vi "GetAllMethodsTypesForClass.vi"(0 "ClassWriterNative":refnum<class "ClassWriterNative.lvclass">, 5 "ClassItemRefIn":refnum<vi>, 11 "error in":errorcluster) -> (2 "MethodTemplatePathOut":path, 3 "DesignPattern":T4[](array[typedef]), 4 "NormalMethods":T2[](array[typedef]), 6 "OverrideMethods":T2[](array[typedef]), 8 "PropertyMethods":T2[](array[typedef]), 10 "ConnectorPaneHeight":i32[](array[numeric]), 13 "TemplateSettings":T1, 14 "PropertyNodeMethods":T2[](array[typedef]), 15 "error out":errorcluster)   [LabVIEW 2012, in "ClassWriterNative.lvclass"]
uses:
  <resource>/Framework/Providers/Open_GDS/ClassProviders/Provider_LvNativeClass/ClassWriterNative_class/ClassWriterNative.lvclass
  <resource>/Framework/Providers/Open_GDS/ClassProviders/Provider_LvNativeClass/ClassWriterNative_class/MethodInfo.ctl
  <resource>/Framework/Providers/Open_GDS/ClassProviders/Provider_LvNativeClass/ClassWriterNative_class/MethodType.ctl
  <resource>/Framework/Providers/Open_GDS/ClassProviders/Common/LvClass_class/GDSLvClass_PlugIn.ctl
  <resource>/Framework/Providers/Open_GDS/ClassProviders/Common/LvClass_class/GDSLvClass_PlugInTypes.ctl
  <resource>/Framework/Providers/Open_GDS/ClassProviders/Provider_BaseClassInterface/ClassWriter_class/TemplateSettings.ctl
  <resource>/Framework/Providers/Open_GDS/ClassProviders/Provider_BaseClassInterface/BaseProvider_SubVIs/BaseProvider_PlugInManagerActions.ctl
  <resource>/Framework/Providers/Open_GDS/ClassProviders/Provider_BaseClassInterface/ClassWriter_class/ClassWriter.lvclass
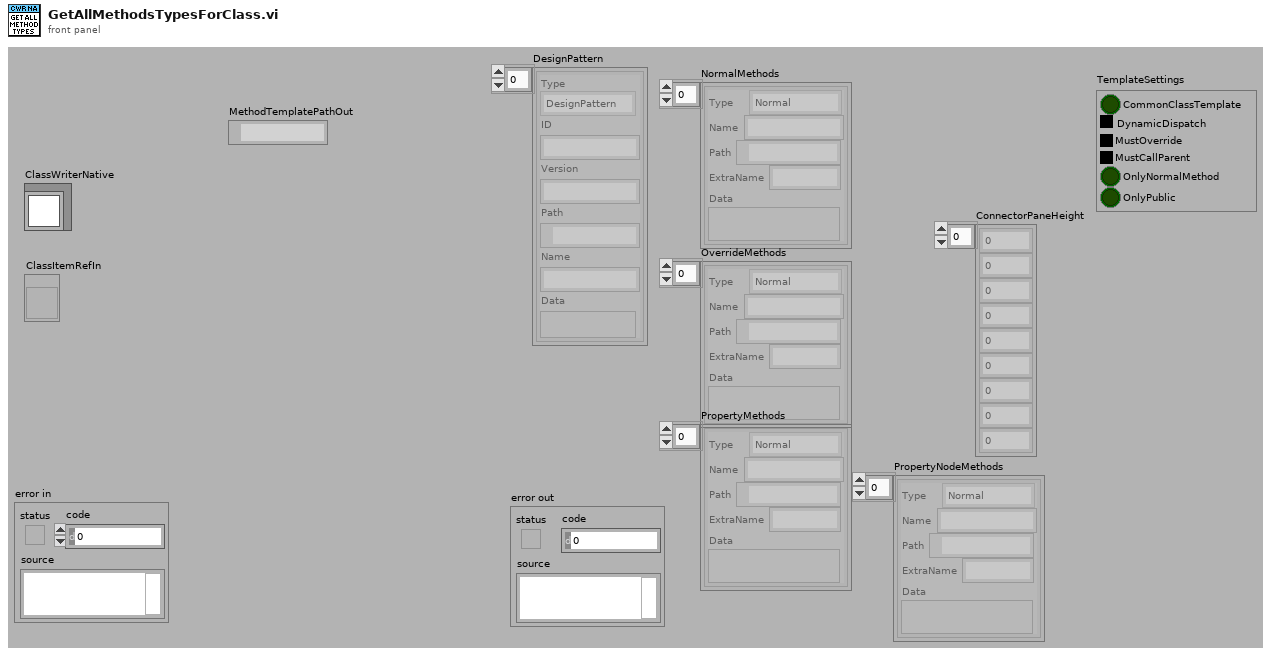
[diagram p1: front panel]
types:
  T1 = typedef "ClassWriter.lvclass/TemplateSettings.ctl" = cluster{"CommonClassTemplate":bool, "DynamicDispatch":enum8{"False", "True", "Mixed"}, "MustOverride":enum8{"False", "True", "Mixed"}, "MustCallParent":enum8{"False", "True", "Mixed"}, "OnlyNormalMethod":bool, "OnlyPublic":bool}
  T2 = typedef "ClassWriterNative.lvclass/MethodInfo.ctl" = cluster{"Type":T3, "Name":string, "Path":path, "ExtraName":string, "Data":variant}
  T3 = typedef "ClassWriterNative.lvclass/MethodType.ctl" = enum16{"Normal", "MethodPlugIn", "DesignPattern", "AF-Method"}
  T4 = typedef "GDSLvClass_PlugIn.ctl" = cluster{"Type":T5, "ID":string, "Version":string, "Path":path, "Name":string, "Data":variant}
  T5 = typedef "GDSLvClass_PlugInTypes.ctl" = enum16{"DesignPattern", "MethodTypes"}
  T6 = typedef "GDSLvCLass_ClassSettingsType.ctl" = cluster{"ClassProviderName":string, "ClassTemplateUsed":string, "ClassTemplateVersion":string, "ClassDescription":string, "PlugIns":T4[], "ConnectorPanePattern":string}
  T7 = typedef "BaseProvider_PlugInManagerActions.ctl" = enum16{"GetPluginsMethods", "ExecutePlugIn"}
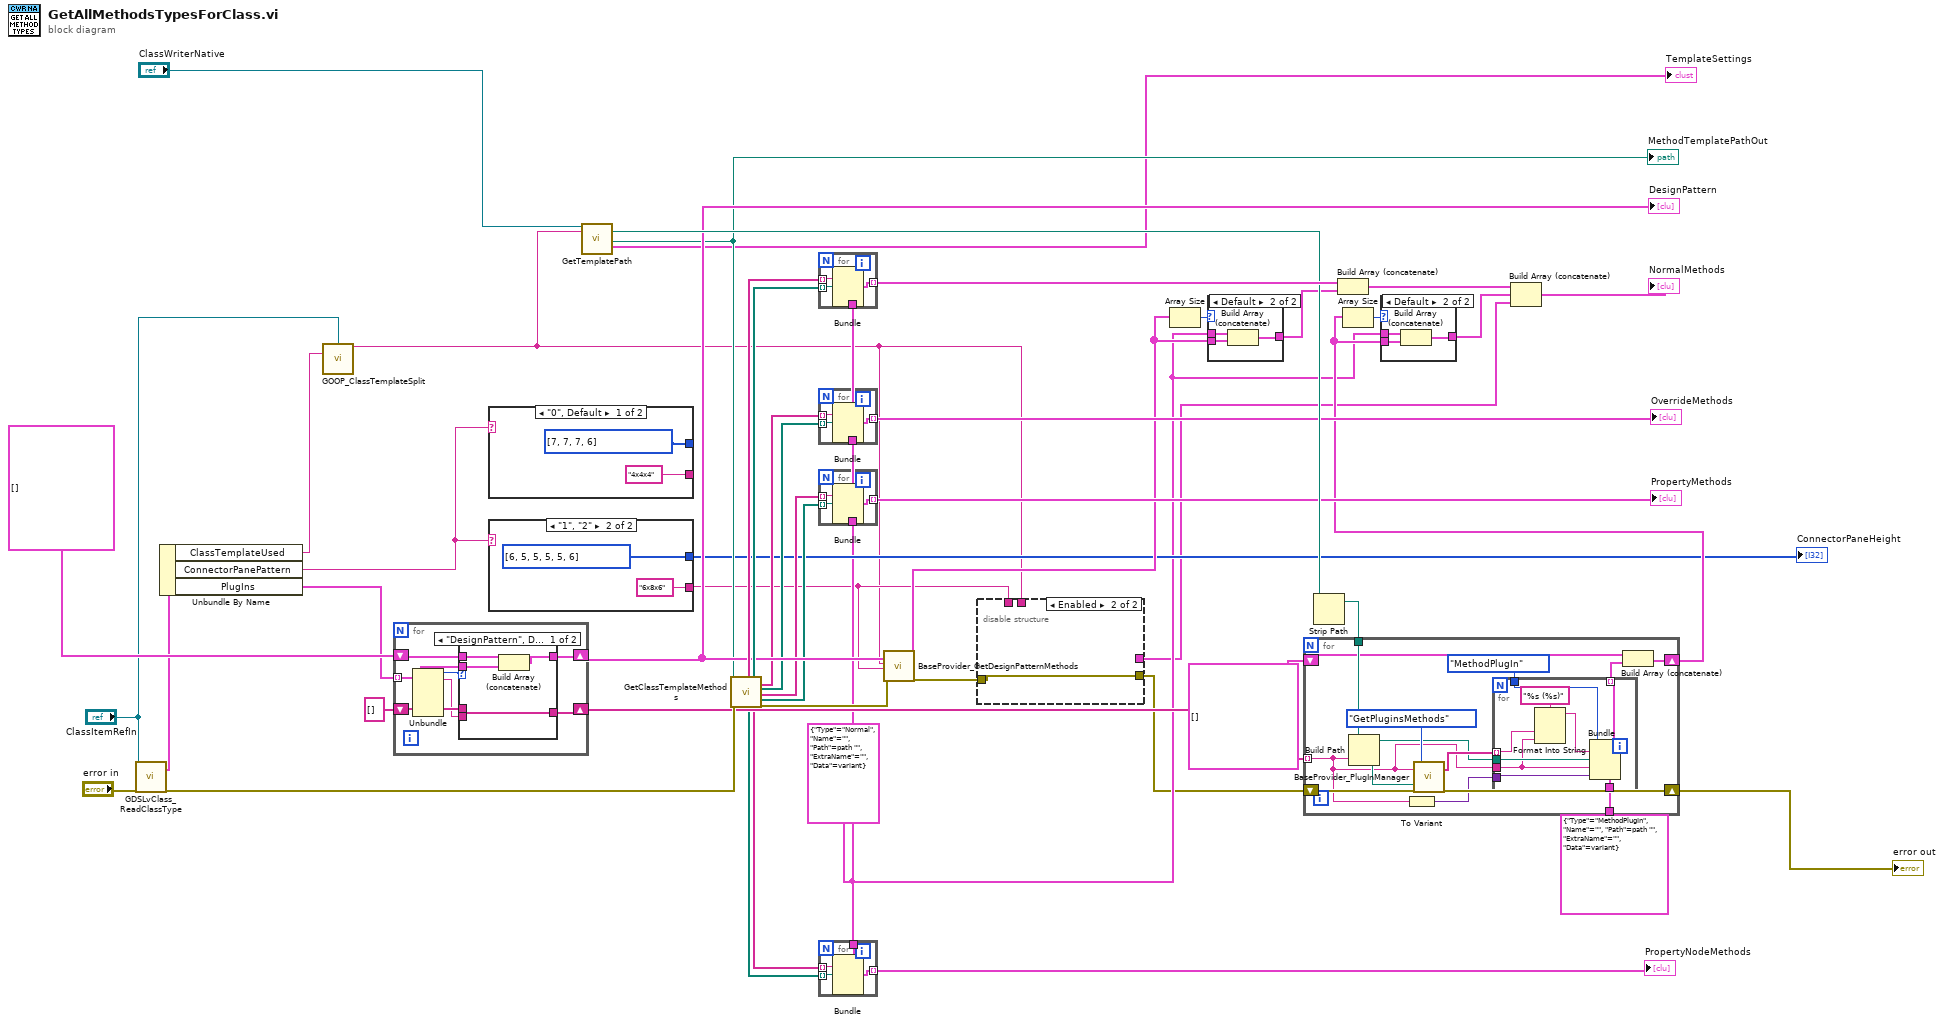
[diagram p0: block diagram]
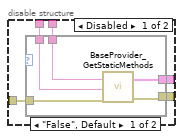
[diagram p2: hidden frame]
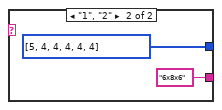
[diagram p4: hidden frame]
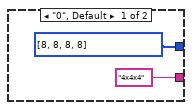
[diagram p5: hidden frame]
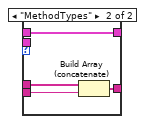
[diagram p8: hidden frame]
diagram:
  w10 = T2 {"Type"=enum."Normal", "Name"="", "Path"=path "", "ExtraName"="", "Data"=variant} ("Cluster")
  n1 = call <resource>:"GDSLvClass_ReadClassType.vi"("Class Refnum In"="ClassItemRefIn", "error in (no error)"="error in") -> ("ClassSettings"=w33:T6, "error out"=w46:errorcluster)  [unwired: 15 in, 1 out]
  n2 = Unbundle By Name(w33) -> ("ClassTemplateUsed"=w13:string, "ConnectorPanePattern"=w12:string, "PlugIns"=w35:T4[])
  n3 = call <resource>:"GOOP_ClassTemplateSplit.vi"("ClassItemRefIn"="ClassItemRefIn", "FullClassTemplate"=w13) -> ("StandardTemplate"=w2:string)  [unwired: 12 in, 1 out]
  n4 = for {
    tunnel: w35 -> [w48] mode=indexing
    shift-right: [w52] -> w41
    shift-left: string[] [] -> [w53]
    shift-right: [w49] -> w37
    shift-left: T4[] [] -> [w50]
    n5 = Unbundle(w48) -> ("Type"=w54:T5, "ID"=w51:string)  [unwired: 4 out]
    n6 = case shown="\"DesignPattern\", Default" w54 {
      tunnel: w53 -> [w58 w62]
      tunnel: [w58 w61] -> w52
      tunnel: w51 -> [_ w60]
      tunnel: w50 -> [w57 w59]
      tunnel: [w56 w59] -> w49
      tunnel: w48 -> [w55 _]
      frame "DesignPattern", Default {
        n7 = Build Array (concatenate)(w57, w55) -> (w56:T4[])
      }
      frame "MethodTypes" {
        n8 = Build Array (concatenate)(w62, w60) -> (w61:string[])
      }
    }
  }
  "DesignPattern" <- w37
  n9 = case shown="\"0\", Default" w12 {
    tunnel: ["4x4x4" "6x8x6"] -> _
    tunnel: [i32[] [7, 7, 7, 6] ("ConnectorPaneHeight") i32[] [5, 4, 4, 4, 4, 4] ("ConnectorPaneHeight")] -> _
    frame "0", Default {
    }
    frame "1", "2" {
    }
  }
  n10 = case shown="\"1\", \"2\"" w12 {
    tunnel: ["4x4x4" "6x8x6"] -> w3
    tunnel: [i32[] [8, 8, 8, 8] ("ConnectorPaneHeight") i32[] [6, 5, 5, 5, 5, 6] ("ConnectorPaneHeight")] -> w14
    frame "0", Default {
    }
    frame "1", "2" {
    }
  }
  "ConnectorPaneHeight" <- w14
  n11 = call-dynamic "GetTemplatePath.vi"("reference in"="ClassWriterNative", "ClassTemplateSubDirectory"=w2) -> ("FolderPathOut"=w39:path, "MethodTemplatePathOut"=w24:path, "TemplateSettings"=→"TemplateSettings":T1)  [unwired: 13 in, 2 out]
  "MethodTemplatePathOut" <- w24
  n12 = call <resource>:"GetClassTemplateMethods.vi"("MethodTemplatePath"=w24, "error in"=w46) -> ("NormalMethodNames"=w42:string[], "PropertyNodeMethodPaths"=w8:path[], "NormalMethodPaths"=w43:path[], "PropertyNodeMethodNames"=w9:string[], "OverrideMethodNames"=w32:string[], "OverrideMethodPaths"=w31:path[], "PropertyMethodNames"=w29:string[], "PropertyMethodPaths"=w28:path[], "error out"=w47:errorcluster)  [unwired: 9 in]
  n13 = for {
    tunnel: w42 -> [w73] mode=indexing
    tunnel: w43 -> [w72] mode=indexing
    tunnel: w10 -> [w74]
    tunnel: [w71] -> w44 mode=indexing
    n14 = Bundle(cluster=w74, "Name"=w73, "Path"=w72) -> (w71:T2)  [unwired: 3 in]
  }
  n15 = for {
    tunnel: w32 -> [w77] mode=indexing
    tunnel: w31 -> [w76] mode=indexing
    tunnel: w10 -> [w78]
    tunnel: [w75] -> w30 mode=indexing
    n16 = Bundle(cluster=w78, "Name"=w77, "Path"=w76) -> (w75:T2)  [unwired: 3 in]
  }
  "OverrideMethods" <- w30
  n17 = for {
    tunnel: w29 -> [w81] mode=indexing
    tunnel: w28 -> [w80] mode=indexing
    tunnel: w10 -> [w82]
    tunnel: [w79] -> w27 mode=indexing
    n18 = Bundle(cluster=w82, "Name"=w81, "Path"=w80) -> (w79:T2)  [unwired: 3 in]
  }
  "PropertyMethods" <- w27
  n19 = for {
    tunnel: w9 -> [w85] mode=indexing
    tunnel: w8 -> [w84] mode=indexing
    tunnel: w10 -> [w86]
    tunnel: [w83] -> w7 mode=indexing
    n20 = Bundle(cluster=w86, "Name"=w85, "Path"=w84) -> (w83:T2)  [unwired: 3 in]
  }
  "PropertyNodeMethods" <- w7
  n21 = call <resource>:"BaseProvider_GetDesignPatternMethods.vi"("DesignPattern"=w37, "ClassTemplateName"=w2, "ConnectorPaneSettings"=w3, "error in"=w47) -> ("NormalMethods"=w16:T2[], "error out"=w6:errorcluster)  [unwired: 14 in]
  n22 = disable-structure shown="Enabled" {
    disable-tunnel: w6 -> [w91 w98]
    disable-tunnel: [w90 w98] -> w5
    disable-tunnel: [w89 _] -> w4
    disable-tunnel: w3 -> [w88 _]
    disable-tunnel: w2 -> [w87 _]
    frame Disabled {
      n23 = case shown="\"False\", Default" {
        selector: _ -> [_ _]
        tunnel: w91 -> [w96 w97]
        tunnel: [w95 w97] -> w90
        tunnel: [w94 _] -> w89
        tunnel: w88 -> [w93 _]
        tunnel: w87 -> [w92 _]
        frame "False", Default {
          n24 = call <resource>:"BaseProvider_GetStaticMethods.vi"("ClassTemplateName"=w92, "ConnectorPaneSettings"=w93, "error in"=w96) -> ("NormalMethods"=w94:T2[], "error out"=w95:errorcluster)  [unwired: 15 in]
        }
        frame "True" {
        }
      }
    }
    frame Enabled {
    }
  }
  n25 = Array Size(array=w16) -> (size(s)=w26:i32)
  n26 = case shown="Default" w26 {
    tunnel: w16 -> [w99 w102]
    tunnel: [w99 w101] -> w25
    tunnel: w10 -> [_ w100]
    frame 0 {
    }
    frame Default {
      n27 = Build Array (concatenate)(w100, w102) -> (w101:T2[])
    }
  }
  n28 = Strip Path(path=w39) -> (stripped path=w40:path)  [unwired: 1 out]
  n29 = for {
    shift-right: [w114] -> w45
    shift-left: w5 -> [w113]
    tunnel: w41 -> [w103] mode=indexing
    tunnel: w40 -> [w112]
    shift-right: [w110] -> w17
    shift-left: T2[] [] -> [w111]
    tunnel: T2 {"Type"=enum."MethodPlugIn", "Name"="", "Path"=path "", "ExtraName"="", "Data"=variant} ("Cluster") -> [w109]
    n30 = Build Path(base path=w112, name or relative path=w103) -> (appended path=w105:path)
    n31 = To Variant(anything=w103) -> (Variant=w104:variant)
    n32 = call <resource>:"BaseProvider_PlugInManager.vi"("PlugInName"=w103, "PlugInPath"=w105, "error in (no error)"=w113, "Action"=BaseProvider_PlugInManagerActions."GetPluginsMethods") -> ("MethodsTypes"=w108:string[], "error out"=w114:errorcluster)  [unwired: 14 in]
    n33 = for {
      tunnel: w108 -> [w118] mode=indexing
      tunnel: w109 -> [w124]
      tunnel: [w123] -> w107 mode=indexing
      tunnel: w104 -> [w120]
      tunnel: MethodType."MethodPlugIn" ("Type") -> [w122]
      tunnel: w105 -> [w121]
      tunnel: w103 -> [w117]
      n34 = Format Into String(format string="%s (%s)", w118, w117) -> (resulting string=w116:string)  [unwired: 2 in, 1 out]
      n35 = Bundle(cluster=w124, "Type"=w122, "Name"=w116, "Path"=w121, "ExtraName"=w117, "Data"=w120) -> (w123:T2)
    }
    n36 = Build Array (concatenate)(w111, w107) -> (w110:T2[])
  }
  "error out" <- w45
  n37 = Build Array (concatenate)(w44, w25) -> (w22:T2[])
  n38 = Array Size(array=w17) -> (size(s)=w23:i32)
  n39 = case shown="Default" w23 {
    tunnel: [w125 w128] -> w18
    tunnel: w17 -> [w125 w127]
    tunnel: w10 -> [_ w126]
    frame 0 {
    }
    frame Default {
      n40 = Build Array (concatenate)(w126, w127) -> (w128:T2[])
    }
  }
  n41 = Build Array (concatenate)(w22, w18, w4) -> (→"NormalMethods":T2[])
